vi "Test New File Sink Error Case.vi"(11 "Test Case In":refnum<class "File Sink.lvclass">) -> (0 "error out":errorcluster, 3 "Test Case Out":refnum<class "File Sink.lvclass">)   [LabVIEW 2020, in "File Sink.lvclass"]
uses:
  File Sink.lvclass
  C:/Program Files (x86)/National Instruments/LabVIEW 2020/vi.lib/Astemes/LUnit/Test Case.lvclass
  Source/Sinks/File Sink/File Sink.lvclass/File Sink.ctl
  <vilib>/Astemes/LUnit/Test Case.lvclass/Test Case.ctl
  4993e8ee-a06a-463a-9684-69129f64d5ce.vi
  <vilib>/Astemes/LUnit/Core/LUnit Test Case/Private/Append Pass Result.vi
  <vilib>/Astemes/LUnit/Core/LUnit Test Case/Private/Append Fail Result.vi
  4993e8ee-a06a-463a-9684-69129f64d5ce.vi/9c5d11cd-9439-4240-a1ee-d9baace9c924.vi
  <vilib>/Astemes/LUnit/Core/LUnit Test Case/Private/Run In UI.vi
  File Sink.lvclass/File Sink.ctl
  Source/Sinks/File Sink/File Sink.lvclass
  <vilib>/Astemes/LUnit/Test Case.lvclass
  C:/Program Files (x86)/National Instruments/LabVIEW 2020/vi.lib/Astemes/LUnit/LUnit Runnable.lvclass
  C:/Users/hughe_cx/Documents/05_repos/LVLog/Testing/File Sink/File Sink.lvclass
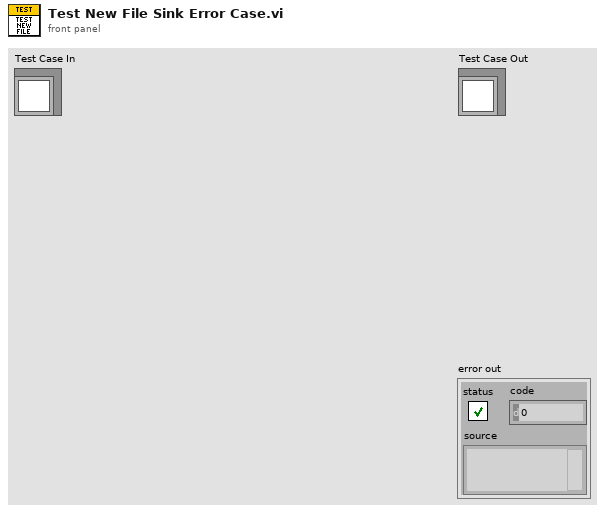
[diagram p1: front panel]
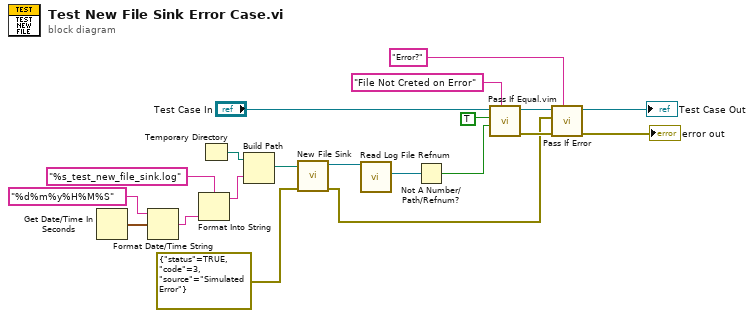
[diagram p0: block diagram]
diagram:
  n1 = Get Date/Time In Seconds() -> (seconds since 1Jan1904=w7:timestamp)
  n2 = Format Date/Time String(time format string (%c)="%d%m%y%H%M%S", seconds (now)=w7) -> (date/time string=w5:string)  [unwired: 1 in]
  n3 = Format Into String(format string="%s_test_new_file_sink.log", w5) -> (resulting string=w8:string)  [unwired: 2 in, 1 out]
  n4 = Temporary Directory() -> (w10:path)
  n5 = Build Path(base path=w10, name or relative path=w8) -> (appended path=w11:path)
  n6 = call "New File Sink.vi"("error in (no error)"=errorcluster {"status"=TRUE, "code"=3, "source"="Simulated Error"}, "File Path"=w11) -> ("error out"=w3:errorcluster, "File Sink out"=w19:refnum<class "File Sink.lvclass">)  [unwired: 8 in]
  n7 = call "Read Log File Refnum.vi"("File Sink in"=w19) -> ("Log File Refnum"=w2:refnum<file>)  [unwired: 8 in, 2 out]
  n8 = Not A Number/Path/Refnum?(number/path/refnum=w2) -> (NaN/Path/Refnum?=w1:bool)
  n9 = call "Pass If Equal.vim"("Description"="File Not Creted on Error", "Actual"=w1, "Expected"=TRUE, "LUnit Test Case In"="Test Case In") -> ("error out"=w14:errorcluster, "LUnit Test Case Out"=w16:refnum<class "File Sink.lvclass">)  [unwired: 6 in]
  n10 = call <vilib>:"Pass If Error.vi"("Description"="Error?", "error in (no error)"=w14, "Assert error"=w3, "LUnit Test Case In"=w16) -> ("error out"=→"error out":errorcluster, "LUnit Test Case Out"=→"Test Case Out":refnum<class "File Sink.lvclass">)  [unwired: 6 in]
